vi "robotimageprocessing.vi"(0 "Image In":T1, 7 "error in":errorcluster) -> (20 "Image Out":T1, 21 "Number of Matches (Shape Matching 1)":i32, 22 "Shape Report (Shape Matching 1)":T2(array[cluster]) {"Score" format="%.2f"; "Centroid"."y" format="%.2f"; "Centroid"."x" format="%.2f"}, 23 "Shape Report (calibrated) (Shape Matching 1)":T2(array[cluster]) {"Score" format="%.2f"; "Centroid"."y" format="%.2f"; "Centroid"."x" format="%.2f"}, 27 "error out":errorcluster)   [LabVIEW 2015]
uses:
  <vilib>/vision/Image Controls.llb/IMAQ Image.ctl
  <vilib>/vision/NI_Vision_Development_Module.lvlib
panel:
  out "Image Out 2":T1(plugin-control)
  out "error out 2":errorcluster
  out "file or folder exists?":bool
  in  "Blue or Luma or Val or Inten Range":cluster{"Lower value":i32, "Upper value":i32}={"Lower value"=241, "Upper value"=255}
  in  "Green or Sat Range":cluster{"Lower value":i32, "Upper value":i32}={"Lower value"=238, "Upper value"=255}
  in  "Red or Hue Range":cluster{"Lower value":i32, "Upper value":i32}={"Lower value"=239, "Upper value"=255}
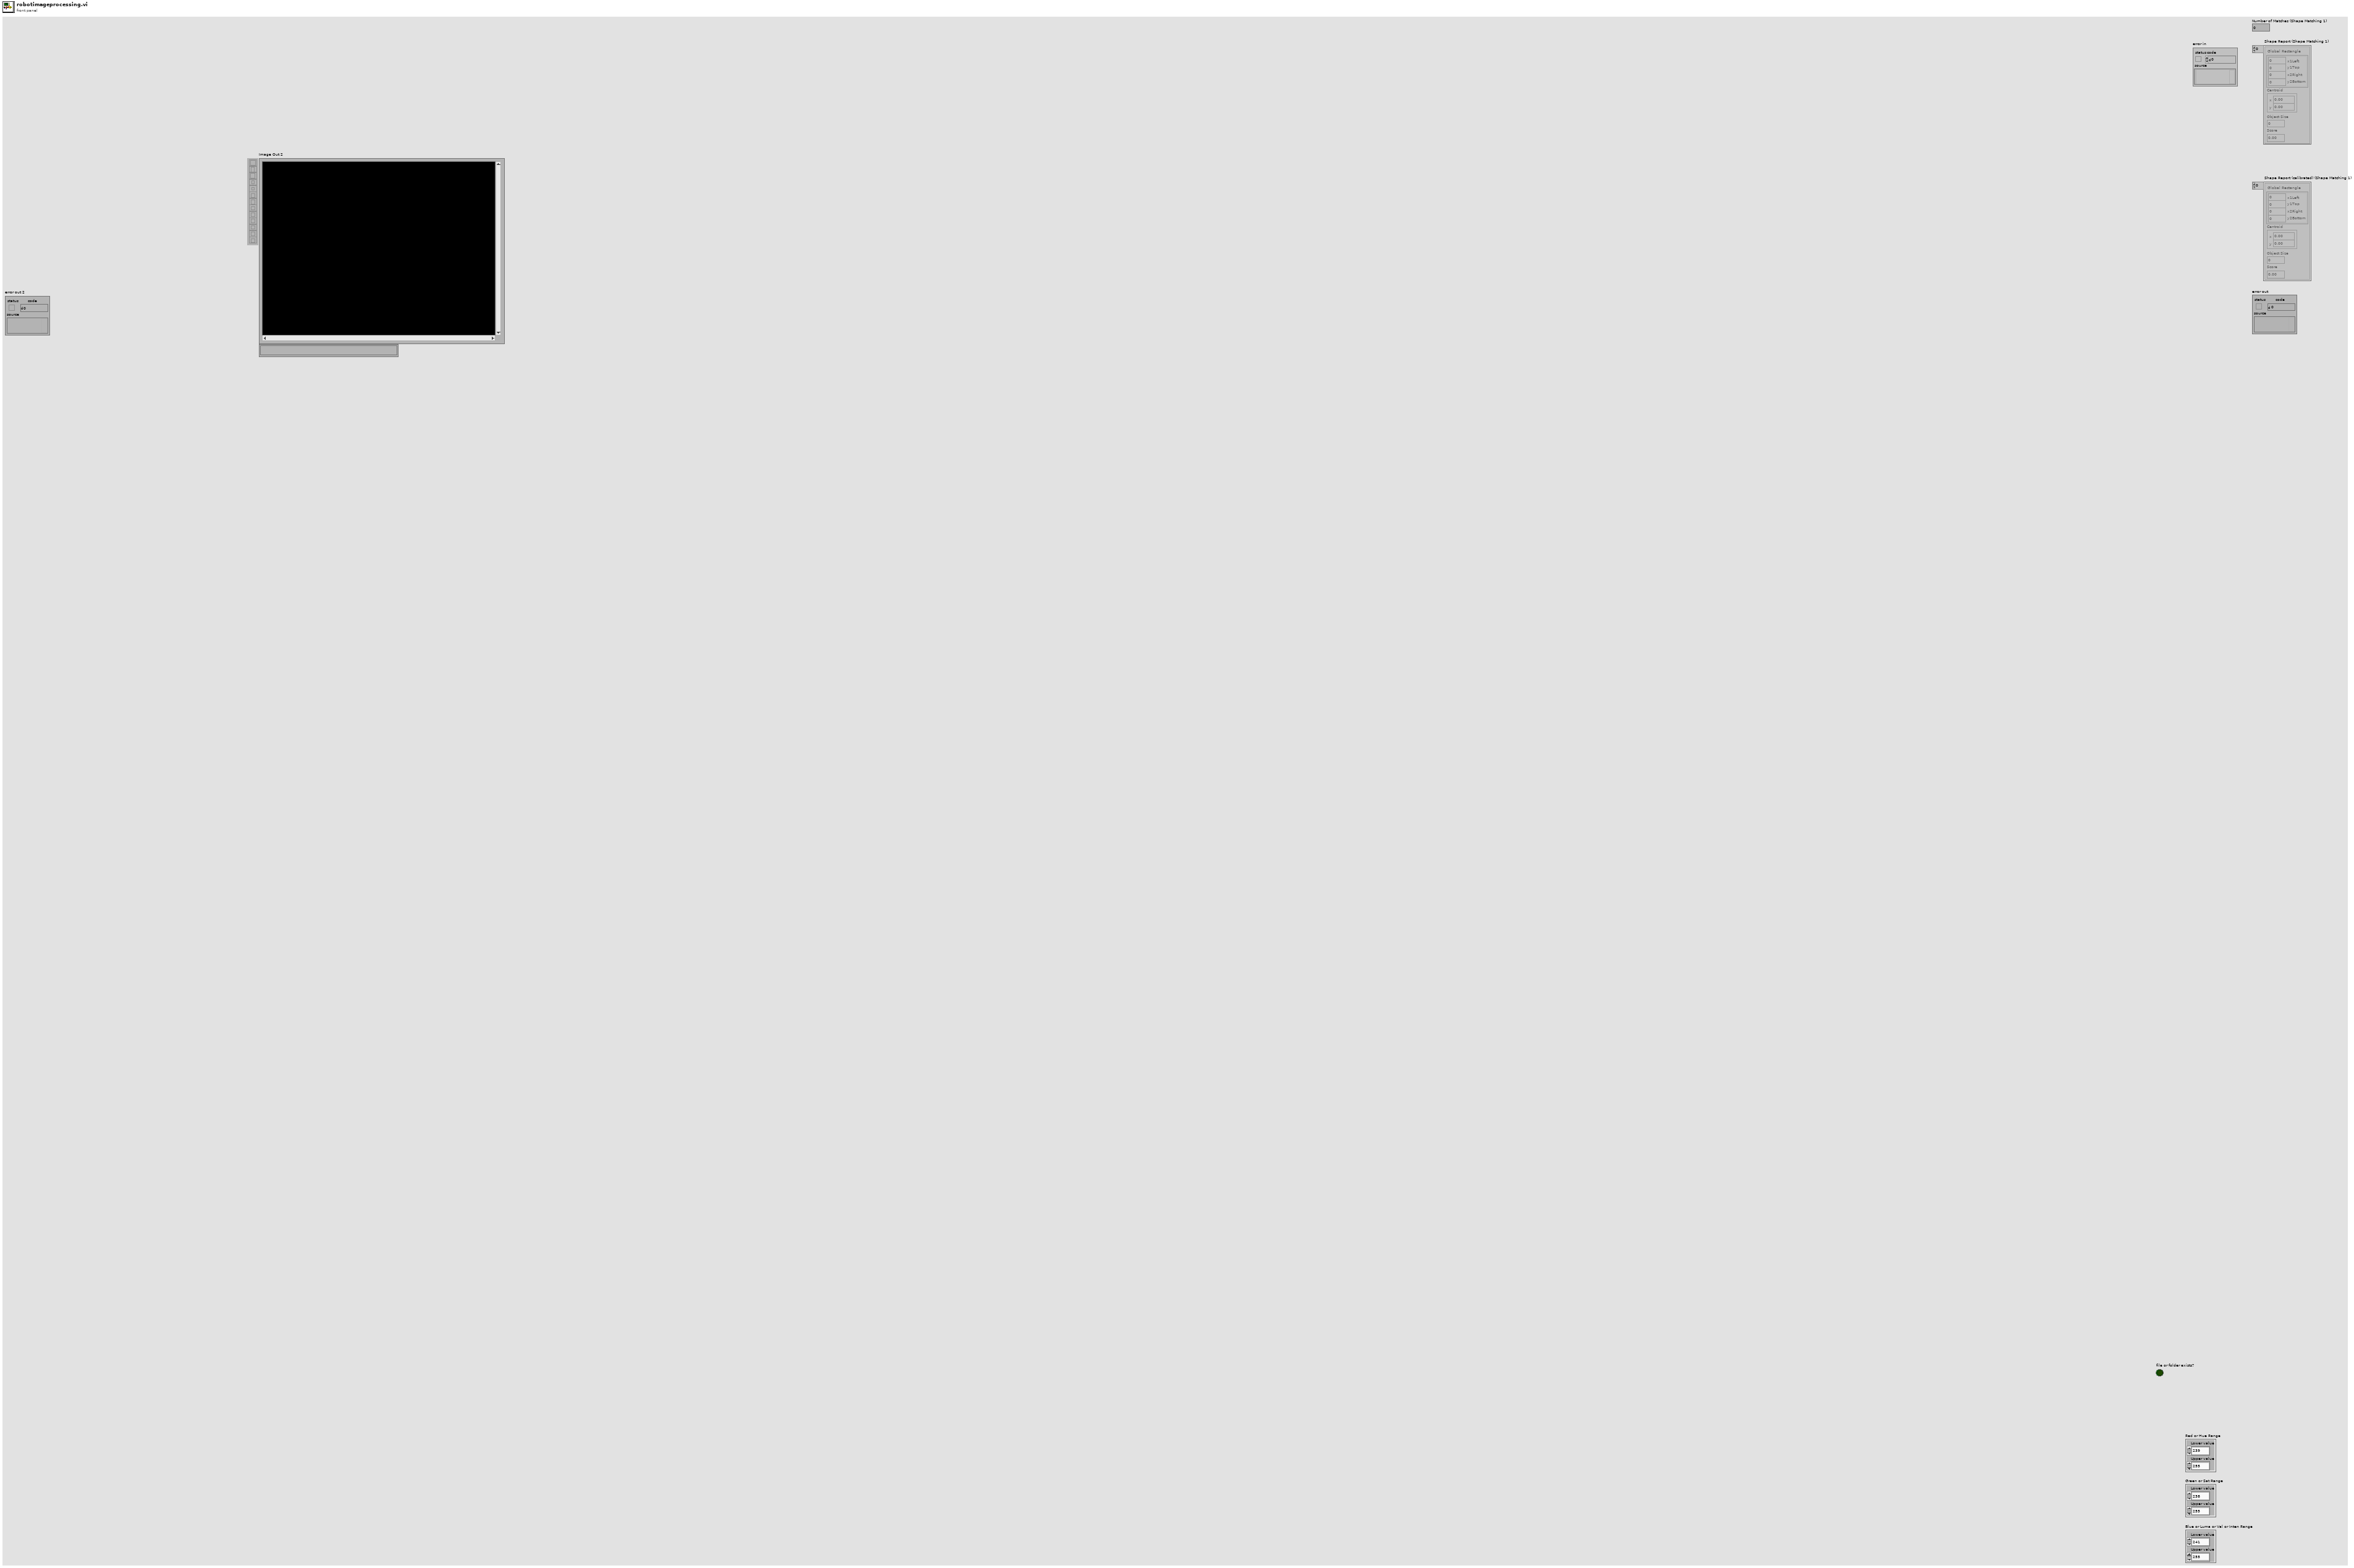
[diagram p1: front panel]
types:
  T1 = typedef "IMAQ Image.ctl" = refnum<image>
  T2 = cluster{"Global Rectangle":cluster{"x1Left":i32, "y1Top":i32, "x2Right":i32, "y2Bottom":i32}, "Centroid":cluster{"x":sgl, "y":sgl}, "Object Size":u32, "Score":dbl}[]
  T3 = enum32{"AutoM", "Close", "Dilate", "Erode", "Gradient", "Gradient out", "Gradient in", "Hit miss", "Open", "PClose", "POpen", "Thick", "Thin"}
  T4 = cluster{"Measurement Parameter":i32, "Range Lower Value":dbl, "Range Upper Value":dbl, "Range":bool, "Measurement Type":bool}[]
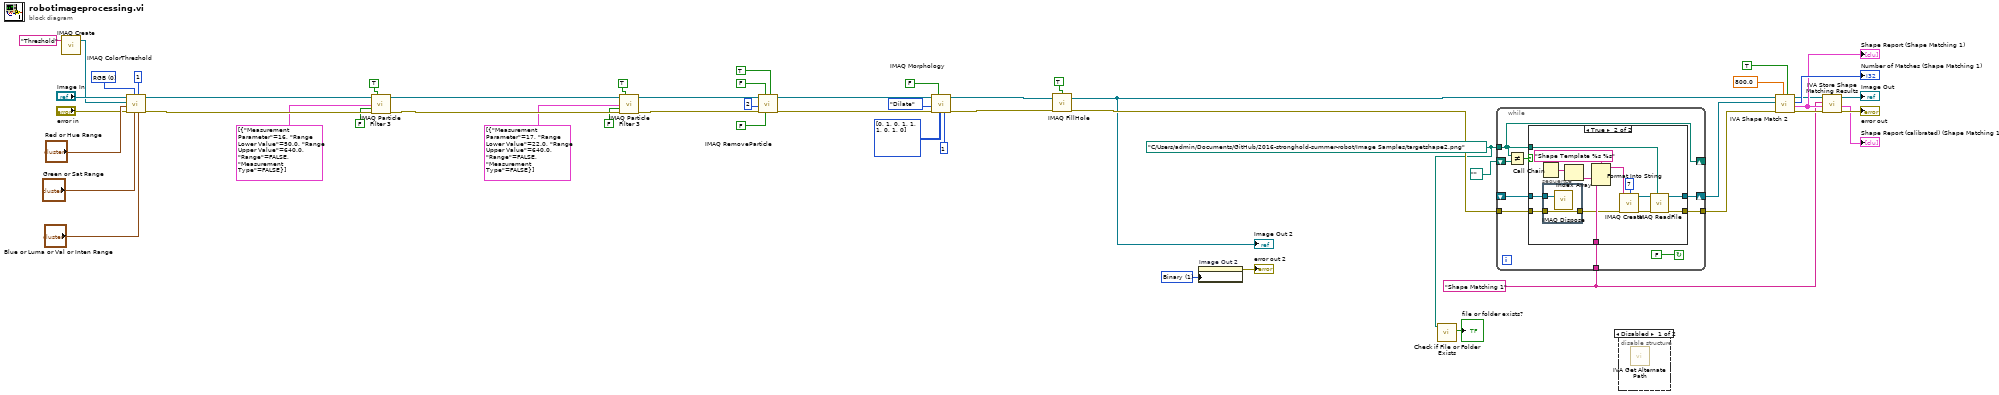
[diagram p0: block diagram]
diagram:
  w3 = u32 1 items=["Grayscale", "Binary", "Gradient", "Rainbow", "Temperature", "User Defined", "Binary 16 Bit", "Gradient 16 Bit", "Rainbow 16 Bit", "Temperature 16 Bit", "User Defined 16 Bit"] ("Palette Type")
  w9 = "Shape Matching 1" ("Step Name")
  w6 = path "C:/Users/admin/Documents/GitHub/2016-stronghold-summer-robot/Image Samples/targetshape2.png" ("Template Path")
  w52 = u16 0 items=["RGB", "HSL", "HSV", "HSI"] ("Color Mode")
  n1 = call "IMAQ Create"("Image Name"="Threshold") -> ("New Image"=w7:T1)  [unwired: 4 in, 1 out]
  n2 = call "IMAQ ColorThreshold"("Blue or Luma or Val or Inten Range"="Blue or Luma or Val or Inten Range", "Replace Value"=1, "Green or Sat Range"="Green or Sat Range", "Color Mode"=w52, "error in (no error)"="error in", "Red or Hue Range"="Red or Hue Range", "Image Dst"=w7, "Image Src"="Image In") -> ("error out"=w46:errorcluster, "Image Dst Out"=w42:T1)  [unwired: 2 out]
  n3 = call "IMAQ Particle Filter 3"("Image Src"=w42, "Connectivity 4/8 (8)"=TRUE, "Selection Values"=T4 [{"Measurement Parameter"=16, "Range Lower Value"=50.0, "Range Upper Value"=640.0, "Range"=FALSE, "Measurement Type"=FALSE}], "Keep/Remove Particles (F)"=FALSE ("Keep/Remove Particles"), "error in (no error)"=w46) -> ("Image Dst Out"=w37:T1, "error out"=w43:errorcluster)  [unwired: 4 in, 5 out]
  n4 = call "IMAQ Particle Filter 3"("Image Src"=w37, "Connectivity 4/8 (8)"=TRUE, "Selection Values"=T4 [{"Measurement Parameter"=17, "Range Lower Value"=22.0, "Range Upper Value"=640.0, "Range"=FALSE, "Measurement Type"=FALSE}], "Keep/Remove Particles (F)"=FALSE ("Keep/Remove Particles"), "error in (no error)"=w43) -> ("Image Dst Out"=w31:T1, "error out"=w38:errorcluster)  [unwired: 4 in, 5 out]
  n5 = call "IMAQ RemoveParticle"("Connectivity 4/8 (8)"=TRUE, "Low Pass/High Pass (Low)"=FALSE, "Square/Hexa (Square)"=FALSE, "error in (no error)"=w38, "Number of Erosion"=2, "Image Src"=w31) -> ("error out"=w30:errorcluster, "Image Dst Out"=w25:T1)  [unwired: 1 in, 3 out]
  n6 = call "IMAQ Morphology"("Number of iterations (1)"=1, "Structuring Element"=i32[][] [[0, 1, 0], [1, 1, 1], [0, 1, 0]], "Square/Hexa (Square)"=FALSE, "error in (no error)"=w30, "Operation"=T3."Dilate", "Image Src"=w25) -> ("error out"=w24:errorcluster, "Image Dst Out"=w22:T1)  [unwired: 1 in, 3 out]
  n7 = call "IMAQ FillHole"("error in (no error)"=w24, "Image Src"=w22, "Connectivity 4/8 (8)"=TRUE) -> ("error out"=w21:errorcluster, "Image Dst Out"=w2:T1)  [unwired: 1 in, 2 out]
  "Image Out 2" <- w2
  n8 = property on="Image Out 2" class="ImageControl"("Palette:Palette Type"=w3) -> (error out=→"error out 2":errorcluster)  [unwired: 2 in, 1 out]
  n9 = call <vilib>:"Check if File or Folder Exists.vi"("path"=w6) -> ("file or folder exists?"=→"file or folder exists?":bool)  [unwired: 8 in, 2 out]
  n10 = while {
    shift-right: [w62] -> w10
    shift-left: _ -> [w61]
    tunnel: [w59] -> w11
    tunnel: w21 -> [w58]
    tunnel: w6 -> [w56]
    tunnel: w9 -> [w57]
    shift-right: [w56] -> _
    shift-left: path "" ("Template Path") -> [w55]
    stop <- FALSE continue-if-true
    n11 = Not Equal?(x=w56, y=w55) -> (x != y?=w54:bool)
    n12 = case shown="True" w54 {
      tunnel: [w64 w75] -> w62
      tunnel: w61 -> [w64 w68]
      tunnel: [w63 w73] -> w59
      tunnel: w58 -> [w63 w67]
      tunnel: w56 -> [_ w65]
      tunnel: w57 -> [_ w69]
      frame False {
      }
      frame True {
        n13 = Call Chain() -> (call chain=w71:string[])
        n14 = stacked-sequence {
          tunnel: w68 -> [w80]
          tunnel: w67 -> [w79]
          tunnel: [w79] -> w66
          frame #0 {
            n15 = call "IMAQ Dispose"("Image"=w80) -> ()  [unwired: 2 in, 4 out]
          }
        }
        n16 = Index Array(array=w71) -> (element=w70:string)  [unwired: 1 in]
        n17 = Format Into String(format string="Shape Template %s %s" ("Image Name"), w70, w69) -> (resulting string=w78:string)  [unwired: 2 in, 1 out]
        n18 = call "IMAQ Create"("Border Size"=7, "Image Name"=w78, "error in (no error)"=w66) -> ("New Image"=w76:T1, "error out"=w74:errorcluster)  [unwired: 1 in, 1 out]
        n19 = call "IMAQ ReadFile"("File Path"=w65, "error in (no error)"=w74, "Image"=w76) -> ("error out"=w73:errorcluster, "Image Out"=w75:T1)  [unwired: 2 in, 5 out]
      }
    }
  }
  n20 = disable-structure shown="Disabled" {
    frame Disabled {
      n21 = call <vilib>:"IVA Get Alternate Path.vi"() -> ()  [unwired: 1 in, 11 out]
    }
    frame Enabled {
    }
  }
  n22 = call <vilib>:"IVA Shape Match 2.vi"("Scale Invariance"=TRUE, "Minimal Score"=800.0, "error in (no error)"=w11, "Template"=w10, "Image Src"=w2) -> ("error out"=w17:errorcluster, "Shape Report"=w15:T2, "Number of Matches"=→"Number of Matches (Shape Matching 1)":i32, "Image Out"=w14:T1)  [unwired: 3 out]
  "Shape Report (Shape Matching 1)" <- w15
  n23 = call <vilib>:"IVA Store Shape Matching Results.vi"("error in (no error)"=w17, "Shape Report"=w15, "Step Name"=w9, "Image in"=w14) -> ("error out"=→"error out":errorcluster, "Shape Report (calibrated)"=→"Shape Report (calibrated) (Shape Matching 1)":T2, "Image dup"=→"Image Out":T1)  [unwired: 5 out]
